vi "20180314.vi"() -> ()   [LabVIEW 2013]
panel:
  out "Waveform Chart":dbl(graph)
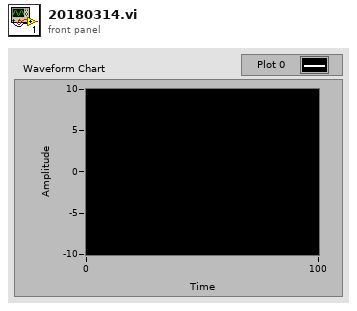
[diagram p1: front panel]
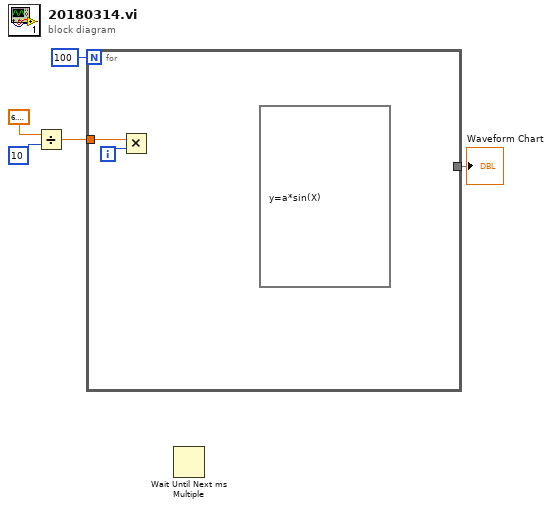
[diagram p0: block diagram]
diagram:
  n1 = Divide(x=6.283185307179586, y=10) -> (x/y=w2:dbl)
  n2 = for {
    N: 100 -> [_]
    tunnel: w2 -> [w7]
    tunnel: [_] -> w1
    i -> [w6]
    n3 = Multiply(x=w7, y=w6) -> ()  [unwired: 1 out]
    n4 = formula code="y=a*sin(X)"() -> ()
  }
  "Waveform Chart" <- w1
  n5 = Wait Until Next ms Multiple() -> ()  [unwired: 1 in, 1 out]
